vi "Write OffensivePlay.vi"(8 "error in (no error)":errorcluster, 10 "Play_v2":refnum<class "Play_v2.lvclass">, 11 "Playbook_v2 in":refnum<class "Playbook_v2.lvclass">) -> (0 "error out":errorcluster, 3 "Playbook_v2 out":refnum<class "Playbook_v2.lvclass">)   [LabVIEW 2023, in "Playbook_v2.lvclass"]
uses:
  Playbook_v2.lvclass
  NewPlays/Play_v2_class/Play_v2.lvclass
  Playbook_v2.lvclass/Playbook_v2.ctl
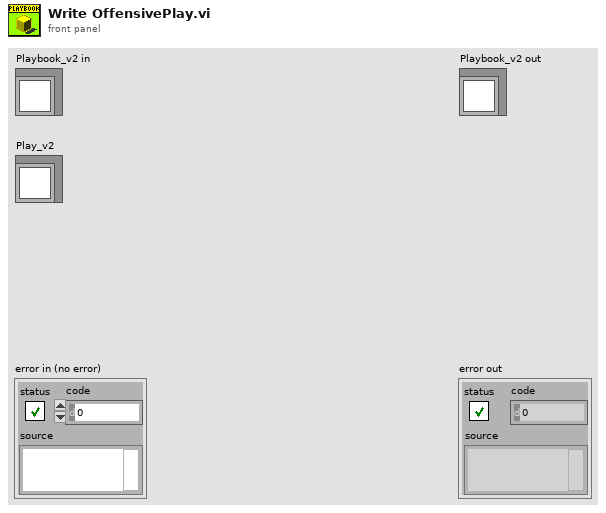
[diagram p1: front panel]
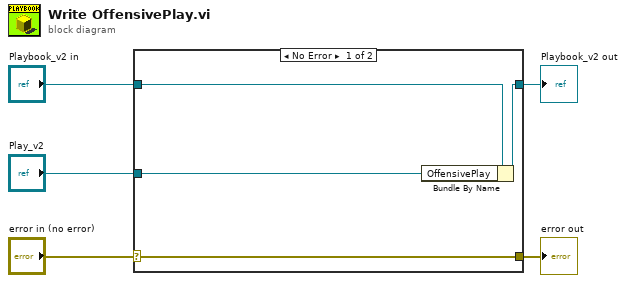
[diagram p0: block diagram]
diagram:
  n1 = case shown="No Error" "error in (no error)" {
    selector: "error in (no error)" -> [w9 w10]
    tunnel: [w9 w10] -> w4
    tunnel: [w7 w11] -> w2
    tunnel: "Playbook_v2 in" -> [w8 w11]
    tunnel: "Play_v2" -> [w6 _]
    frame No Error {
      n2 = Bundle By Name(cluster=w8, "OffensivePlay"=w6) -> (w7:refnum<class "Playbook_v2.lvclass">)
    }
    frame Error {
    }
  }
  "error out" <- w4
  "Playbook_v2 out" <- w2
